vi "Template.vi"(0 "VISA IN":refnum<visa-resource-name>, 5 "error in":errorcluster) -> (14 "VISA Out":refnum<visa-resource-name>, 19 "error out":errorcluster)   [LabVIEW 2018, in "PNA-X.lvlib"]
uses:
  PNA-X.lvlib
panel:
  in  "Amplitude":dbl
  in  "Port":i32=1
  in  "Trace":i32=1
  in  "Window":i32=1
  in  "Channel":i32=1
  in  "Npoints":dbl=1.0
  in  "Span":dbl=10000000.0
  in  "Center":dbl=10000000.0
  in  "Step":dbl=10000000.0
  in  "Stop":dbl=10000000.0
  in  "Start":dbl=10000000.0
  in  "Phase":dbl
  in  "Resolution":dbl=1.0
  in  "IfBw":dbl=1.0
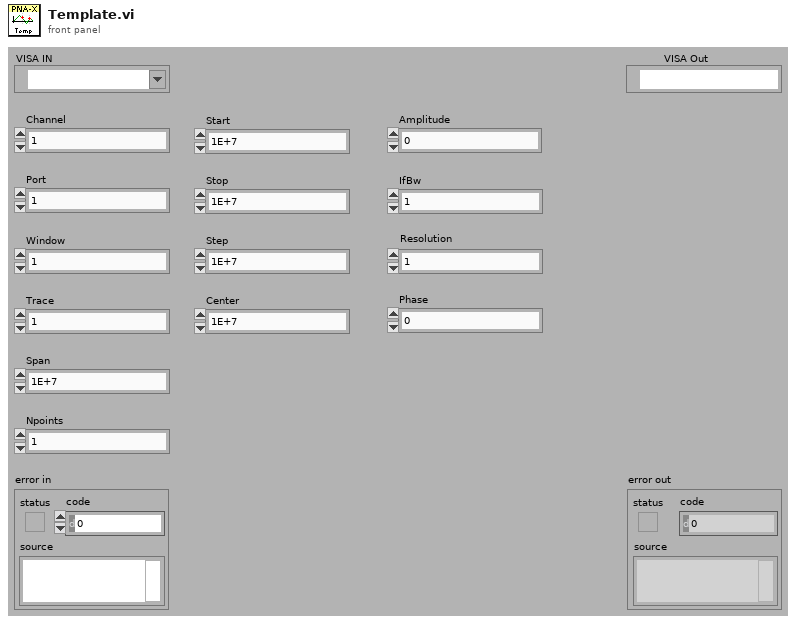
[diagram p1: front panel]
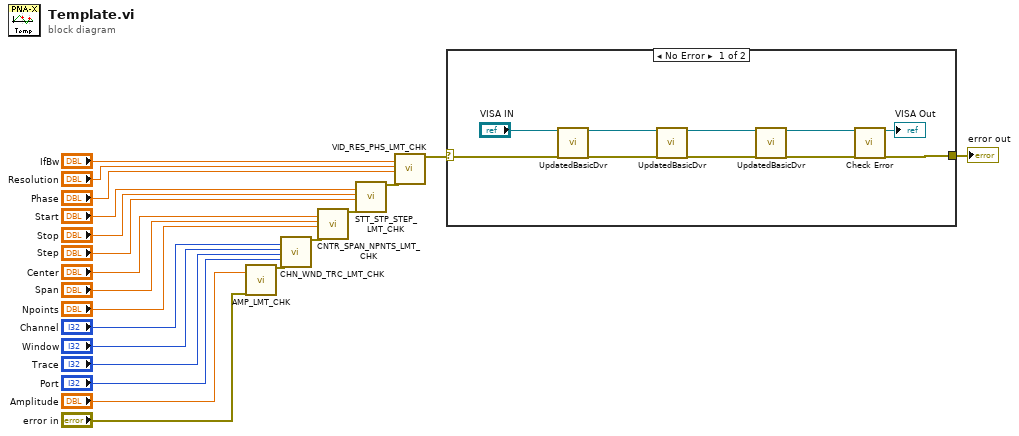
[diagram p0: block diagram]
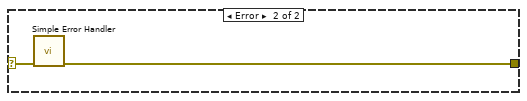
[diagram p2: hidden frame]
diagram:
  n1 = call "AMP_LMT_CHK.vi"("Amplitude"="Amplitude", "error in"="error in") -> ("error out"=w21:errorcluster)  [unwired: 16 in, 1 out]
  n2 = call "CHN_WND_TRC_LMT_CHK.vi"("Channel"="Channel", "Window"="Window", "Trace"="Trace", "Port"="Port", "error in"=w21) -> ("error out"=w20:errorcluster)  [unwired: 10 in, 4 out]
  n3 = call "CNTR_SPAN_NPNTS_LMT_CHK.vi"("Center"="Center", "Span"="Span", "Npoints"="Npoints", "error in"=w20) -> ("error out"=w19:errorcluster)  [unwired: 12 in, 3 out]
  n4 = call "STT_STP_STEP_LMT_CHK.vi"("Start"="Start", "Stop"="Stop", "Step"="Step", "error in"=w19) -> ("error out"=w17:errorcluster)  [unwired: 12 in, 3 out]
  n5 = call "VID_RES_PHS_LMT_CHK.vi"("IF"="IfBw", "Resolution"="Resolution", "Phase"="Phase", "error in"=w17) -> ("error out"=w2:errorcluster)  [unwired: 11 in, 4 out]
  n6 = case shown="No Error" w2 {
    selector: w2 -> [w29 w33]
    tunnel: [w31 w32] -> w1
    frame No Error {
      n7 = call "UpdatedBasicDvr.vi"("VISA IN"="VISA IN", "error in"=w29) -> ("VISA Out"=w24:refnum<visa-resource-name>, "error out"=w28:errorcluster)  [unwired: 16 in]
      n8 = call "UpdatedBasicDvr.vi"("VISA IN"=w24, "error in"=w28) -> ("VISA Out"=w23:refnum<visa-resource-name>, "error out"=w27:errorcluster)  [unwired: 16 in]
      n9 = call "UpdatedBasicDvr.vi"("VISA IN"=w23, "error in"=w27) -> ("VISA Out"=w22:refnum<visa-resource-name>, "error out"=w26:errorcluster)  [unwired: 16 in]
      n10 = call "Check Error.vi"("VISA Resource Name"=w22, "error in (no error)"=w26) -> ("dup VISA session"=→"VISA Out":refnum<visa-resource-name>, "error out"=w31:errorcluster)  [unwired: 16 in]
    }
    frame Error {
      n11 = call <vilib>:"Simple Error Handler.vi"("error in (no error)"=w33) -> ("error out"=w32:errorcluster)  [unwired: 4 in, 4 out]
    }
  }
  "error out" <- w1
